vi "S4GUI_003.vi"(7 "Tab ObsEng":enum32{"Obs", "CCD modes", "Guider", "Eng"}(tab)) -> ()   [LabVIEW 2018] (continued)
      n64 = property on="Project ID" class="Str"(error in=w86, "Value"="" ("Observer"), "Text.BGColor"=u32 16448250) -> ()  [unwired: 1 in, 2 out]
      n65 = property on="SendExpose" class="Bool (strict)"(error in=w86, "Value"=TRUE ("ExtSync")) -> ()  [unwired: 1 in, 2 out]
      n66 = property on="suffix alert" class="Str"(error in=w86, "Text.BGColor"=u32 16711680, "Text.TextColor"=u32 16776722) -> ()  [unwired: 1 in, 2 out]
      n67 = property on="Object_dflat" class="Str"(error in=w86, "DisabledEnum"=w95) -> ()  [unwired: 1 in, 2 out]
      n68 = property on="Object_zero" class="Str"(error in=w86, "DisabledEnum"=w95) -> ()  [unwired: 1 in, 2 out]
      n69 = property on="Object_sflat" class="Str"(error in=w86, "DisabledEnum"=w95) -> ()  [unwired: 1 in, 2 out]
      n70 = local write "GUIDER"(FALSE ("GUIDER")) -> ()
      n71 = property on="Exptime ch1" class="DigNum (strict)"("Value"=w72) -> ()  [unwired: 2 in, 2 out]
      n72 = property on="Exptime ch2" class="DigNum (strict)"("Value"=w72) -> ()  [unwired: 2 in, 2 out]
      n73 = property on="Exptime ch3" class="DigNum (strict)"("Value"=w72) -> ()  [unwired: 2 in, 2 out]
      n74 = property on="Exptime ch4" class="DigNum (strict)"("Value"=w72) -> ()  [unwired: 2 in, 2 out]
      n75 = property on="dark suffix" class="Str"(error in=w82, "Text.BGColor"=u32 16448250) -> ()  [unwired: 1 in, 2 out]
      n76 = property on="object suffix" class="Str"(error in=w82, "Text.BGColor"=u32 16448250) -> (error out=w76:errorcluster)  [unwired: 1 in, 1 out]
      n77 = property on="dflat suffix" class="Str"(error in=w82, "Text.BGColor"=u32 16448250) -> ()  [unwired: 1 in, 2 out]
      n78 = property on="SET Temp message" class="Bool (strict)"(error in=w76, "Value"=TRUE ("SET Temp message")) -> (error out=w71:errorcluster)  [unwired: 1 in, 1 out]
      n79 = local write "TEST Comments"("Acquisition for testing purposes" ("TEST Comments")) -> ()
      n80 = local write "test suffix"("test" ("test suffix")) -> ()
      n81 = local write "Object_test"("TEST OBJECT" ("Object_test")) -> ()
      n82 = property on="sflat suffix" class="Str"(error in=w76, "Text.BGColor"=u32 16448250) -> ()  [unwired: 1 in, 2 out]
      n83 = property on="zero suffix" class="Str"(error in=w76, "Text.BGColor"=u32 16448250) -> ()  [unwired: 1 in, 2 out]
      n84 = property on="focus suffix" class="Str"(error in=w76, "Text.BGColor"=u32 16448250) -> ()  [unwired: 1 in, 2 out]
      "suffix alert" <- "Invalid char!" ("suffix alert")
      "FT warning" <- "" ("FT warning")
    }
    frame #4 {
      w97 = u32 1 ("# Cycles")
      n85 = local write "# Cycles"(w97) -> ()
      n86 = local write "#cycles ch1"(w97) -> ()
      n87 = local write "#cycles ch2"(w97) -> ()
      n88 = local write "#cycles ch3"(w97) -> ()
      n89 = local write "#cycles ch4"(w97) -> ()
      n90 = local write "Exp ch1"(w97) -> ()
      n91 = local write "Exp ch2"(w97) -> ()
      n92 = local write "Exp ch3"(w97) -> ()
      n93 = local write "Exp ch4"(w97) -> ()
    }
  }
  n94 = disable-structure shown="Enabled" {
    disable-tunnel: "S4ACS_GUI.lvclass" -> [w106 w108]
    disable-tunnel: w5 -> [w105 w107]
    disable-tunnel: [w100 w108] -> w25
    disable-tunnel: [w99 w107] -> w24
    frame Enabled {
      # "Carrega o ultimo filtro escolhido para os 4 canais."
      n95 = local read "Filter1"() -> (w104:u8)
      n96 = local read "Filter2"() -> (w103:u8)
      n97 = local read "Filter3"() -> (w102:u8)
      n98 = local read "Filter4"() -> (w101:u8)
      n99 = call-dynamic "LoadFilters.vi"("Filter 4"=w101, "Filter 3"=w102, "error in (no error)"=w105, "Filter 2"=w103, "Filter 1"=w104, "S4GUI in"=w106) -> ("error out"=w99:errorcluster, "S4GUI out"=w100:refnum<class "S4GUI.lvclass">)  [unwired: 4 in]
    }
    frame Disabled {
    }
  }
  n100 = flat-sequence "Indicadores dos canais da parte inferior da tela principal" {
    frame #0 {
      w109 = ""
      "B1" <- w109
      "PA1" <- w109
      "RO1" <- w109
      "G1" <- w109
      "SI2" <- w109
      "PA2" <- w109
      "G2" <- w109
      "B2" <- w109
      "RO2" <- w109
      "EA2" <- w109
      "SI3" <- w109
      "EA3" <- w109
      "PA3" <- w109
      "B3" <- w109
      "G3" <- w109
      "RO3" <- w109
      "SI4" <- w109
      "EA4" <- w109
      "PA4" <- w109
      "B4" <- w109
      "G4" <- w109
      "RO4" <- w109
      "SI1" <- w109
      "EA1" <- w109
    }
  }
  n101 = call-dynamic "Write GUI version.vi"("error in (no error)"=w24, "GUI version"=w22, "S4GUI in"=w25) -> ("error out"=w16:errorcluster, "S4GUI out"=w23:refnum<class "S4GUI.lvclass">)  [unwired: 7 in]
  n102 = property on="Tab Acq Type" class="TabCtl (strict)"(error in=w16, "DisabledEnum"=T12."Disabled and Grayed Out" ("Disabled")) -> (error out=w15:errorcluster)  [unwired: 1 in, 1 out]
  n103 = control-ref of="Current Configuration"() -> (w33:refnum<vi>)
  n104 = control-ref of="Parameters"() -> (w30:refnum<vi>)
  n105 = call-dynamic "Initialize.vi"("error in (no error)"=w15, "S4ACS_GUI in"=w23) -> ("error out"=w14:errorcluster, "S4ACS_GUI out"=w18:refnum<class "S4GUI.lvclass">)  [unwired: 8 in]
  n106 = property on="Tab Acq Type" class="TabCtl (strict)"(error in=w14, "DisabledEnum"=T12."Enabled" ("Disabled")) -> (error out=w13:errorcluster)  [unwired: 1 in, 1 out]
  n107 = property on="Property Node" class="Clust (strict)"(reference=w30, "Top"=230 ("Position:Top")) -> (reference out=w34:refnum<vi>)  [unwired: 1 in, 1 out]
  n108 = property on="Property Node" class="Clust (strict)"(reference=w33, "Top"=230 ("Position:Top")) -> (reference out=w32:refnum<vi>)  [unwired: 1 in, 1 out]
  n109 = call-dynamic "Read TabAcqType index.vi"("error in (no error)"=w13, "S4GUI in"=w18) -> ("error out"=w10:errorcluster, "TabAcqType index"=w17:u32, "S4GUI out"=w11:refnum<class "S4GUI.lvclass">)  [unwired: 7 in]
  n110 = case shown="1" w17 {
    tunnel: [T1."OBJECT" ("Tab Acq Type") T1."TEST" ("Tab Acq Type") T1."DFLAT" ("Tab Acq Type") T1."SFLAT" ("Tab Acq Type") T1."DARK" ("Tab Acq Type") T1."ZERO" ("Tab Acq Type") T1."FOCUS" ("Tab Acq Type")] -> w7
    frame 0, Default {
    }
    frame 1 {
    }
    frame 2 {
    }
    frame 3 {
    }
    frame 4 {
    }
    frame 5 {
    }
    frame 6 {
    }
  }
  n111 = local write "Tab Acq Type"(w7) -> ()
  n112 = Bundle("Parameters"=w34, "Current Configuration"=w32) -> (w31:T13)  [unwired: 1 in]
  n113 = call-dynamic "Write ExpMode.vi"("error in (no error)"=w10, "ExpMode"=w7, "S4GUI in"=w11) -> ("error out"=w9:errorcluster, "S4GUI out"=w8:refnum<class "S4GUI.lvclass">)  [unwired: 7 in]
  n114 = while {
    shift-right: [w135] -> w4
    shift-left: w8 -> [w137]
    shift-right: [w122] -> w2
    shift-left: w9 -> [w118]
    tunnel: w31 -> [w142]
    i -> [w128]
    stop <- w119 stop-if-true
    # "Sufixo do arquivo SEMPRE\nem minúsculas."
    n115 = case shown="\"TEST\"" "Tab Acq Type" {
      tunnel: ["object suffix" "test suffix" "dflat suffix" "sflat suffix" "dark suffix" "zero suffix" "focus suffix"] -> w130
      tunnel: ["OBJECT Comments" "TEST Comments" "DFLAT Comments" "SFLAT Comments" "DARK Comments" "ZERO Comments" "FOCUS Comments"] -> w143
      tunnel: ["OBJECT" "TEST" "FLAT" "FLAT" "DARK" "ZERO" "FOCUS"] -> w140
      tunnel: ["Object_obj" "Object_test" "DOMEFLAT" "SKYFLAT" "Object_dark" "ZERO" "Object_focus"] -> w139
      tunnel: [_ _ _ _ _ _ "Start focus"] -> w127
      tunnel: [_ _ _ _ _ _ "Step focus"] -> w125
      tunnel: [_ _ _ _ _ _ "#steps"] -> w126
      frame "OBJECT", Default {
      }
      frame "TEST" {
      }
      frame "DFLAT" {
      }
      frame "SFLAT" {
      }
      frame "DARK" {
      }
      frame "ZERO" {
      }
      frame "FOCUS" {
      }
    }
    n116 = flat-sequence {
      tunnel: w137 -> [w157]
      tunnel: [w157] -> w117
      tunnel: [w156] -> w134
      frame #0 {
        n117 = case shown="False" "reset max" {
          frame False {
          }
          frame True {
            n118 = local write "loop max(ms)"(u32 0 ("loop max(ms)")) -> ()
          }
        }
        n119 = Tick Count (ms)() -> (millisecond timer value=w156:u32)
      }
    }
    n120 = To Lower Case(string=w130) -> (all lower case string=w129:string)
    n121 = event shown="[57] \"#cycles ch4\": Value Change" {
      selector: _ -> [_ _ _ _ _ _ _ _ _ _ _ _ _ _ _ _ _ _ _ _ _ _ _ _ _ _ _ _ _ _ _ _ _ _ _ _ _ _ _ _ _ _ _ _ _ _ _ _ _ _ _ _ _ _ _ _ _ _ _ _ _ _ _ _ _ _ _ _ _ _ _ _ _ _ _ _ _ _ _ _ _ _ _ _ _ _ _ _ _ _ _ _ _ _ _ _ _ _ _ _ _ _ _ _ _ _ _ _ _ _ _ _ _ _ _ _ _ _ _ _ _ _ _ _ _ _ _ _ _ _ _ _ _ _ _ _ _ _ _ _ _ _ _ _ _]
      dyn-events: _ -> [_ _ _ _ _ _ _ _ _ _ _ _ _ _ _ _ _ _ _ _ _ _ _ _ _ _ _ _ _ _ _ _ _ _ _ _ _ _ _ _ _ _ _ _ _ _ _ _ _ _ _ _ _ _ _ _ _ _ _ _ _ _ _ _ _ _ _ _ _ _ _ _ _ _ _ _ _ _ _ _ _ _ _ _ _ _ _ _ _ _ _ _ _ _ _ _ _ _ _ _ _ _ _ _ _ _ _ _ _ _ _ _ _ _ _ _ _ _ _ _ _ _ _ _ _ _ _ _ _ _ _ _ _ _ _ _ _ _ _ _ _ _ _ _ _]
      timeout: 20 -> [_ _ _ _ _ _ _ _ _ _ _ _ _ _ _ _ _ _ _ _ _ _ _ _ _ _ _ _ _ _ _ _ _ _ _ _ _ _ _ _ _ _ _ _ _ _ _ _ _ _ _ _ _ _ _ _ _ _ _ _ _ _ _ _ _ _ _ _ _ _ _ _ _ _ _ _ _ _ _ _ _ _ _ _ _ _ _ _ _ _ _ _ _ _ _ _ _ _ _ _ _ _ _ _ _ _ _ _ _ _ _ _ _ _ _ _ _ _ _ _ _ _ _ _ _ _ _ _ _ _ _ _ _ _ _ _ _ _ _ _ _ _ _ _ _]
      tunnel: w117 -> [w199 w1995 w2006 w2011 w2016 w2021 w2026 w2031 w2301 w2460 w2490 w2496 w2518 w2540 w2739 w2747 w2826 w2847 w2919 w2990 w3091 w3105 w3246 w3485 w3517 w3549 w3581 w3616 w3651 w3686 w3721 w3724 w3819 w4024 w4085 w4612 w4691 w4763 w4834 w4907 w4958 w4999 w5441 w5447 w5567 w6952 w7095 w7300 w7488 w7752 w7971 w7986 w8197 w8407 w8431 w8455 w8479 w8503 w8518 w8660 w8802 w8931 w8951 w8971 w8991 w9012 w9077 w9142 w9207 w9272 w9309 w9337 w9365 w9394 w9467 w9597 w9631 w9690 w9749 w9808 w9867 w9887 w9914 w9930 w9951 w9981 w10011 w10036 w10077 w10118 w10159 w10200 w10241 w10282 w10323 w10366 w10481 w10591 w10701 w10810 w10820 w10840 w10855 w10870 w10885 w10900 w10915 w10930 w10945 w10976 w11005 w11029 w11071 w11105 w11132 w11155 w11183 w11203 w11218 w11238 w11321 w11649 w11675 w11841 w11861 w11876 w11892 w11912 w11932 w11952 w11972 w11987 w12003 w12023 w12043 w12063 w12083 w12098 w12118 w12138 w12158 w12173 w12193 w12213 w12233]
      tunnel: w118 -> [w198 w1994 w2005 w2010 w2015 w2020 w2025 w2030 w2302 w2458 w2489 w2495 w2517 w2539 w2738 w2746 w2825 w2846 w2918 w2991 w3090 w3097 w3242 w3484 w3516 w3548 w3580 w3615 w3650 w3685 w3720 w3732 w3820 w4023 w4084 w4611 w4690 w4762 w4830 w4906 w4956 w4998 w5397 w5446 w5566 w6951 w7094 w7299 w7487 w7745 w7969 w7985 w8195 w8406 w8430 w8454 w8478 w8502 w8517 w8658 w8801 w8932 w8952 w8972 w8992 w9011 w9076 w9141 w9206 w9270 w9307 w9335 w9363 w9393 w9466 w9596 w9630 w9689 w9748 w9807 w9866 w9886 w9913 w9929 w9950 w9980 w10010 w10035 w10076 w10117 w10158 w10199 w10240 w10281 w10322 w10365 w10480 w10590 w10700 w10809 w10819 w10839 w10854 w10869 w10884 w10899 w10914 w10929 w10944 w10975 w11004 w11028 w11070 w11104 w11131 w11154 w11182 w11202 w11217 w11237 w11322 w11648 w11674 w11840 w11860 w11875 w11891 w11911 w11931 w11951 w11971 w11986 w12002 w12022 w12042 w12062 w12082 w12097 w12117 w12137 w12157 w12172 w12192 w12212 w12232]
      tunnel: [w195 w1993 w2003 w2007 w2012 w2017 w2022 w2027 w2264 w2452 w2477 w2497 w2519 w2541 w2726 w2764 w2825 w2864 w2936 w3008 w3077 w3103 w3244 w3395 w3503 w3535 w3567 w3606 w3641 w3676 w3711 w3732 w3740 w3942 w4072 w4531 w4688 w4760 w4825 w4904 w4959 w4993 w5400 w5443 w5534 w7009 w7088 w7293 w7499 w7746 w7970 w7978 w8183 w8329 w8413 w8438 w8462 w8486 w8504 w8647 w8787 w8930 w8950 w8970 w8990 w9010 w9075 w9140 w9205 w9271 w9308 w9336 w9364 w9398 w9471 w9598 w9629 w9688 w9747 w9806 w9865 w9885 w9912 w9928 w9949 w9979 w10009 w10038 w10079 w10120 w10161 w10202 w10243 w10284 w10325 w10364 w10479 w10589 w10699 w10806 w10818 w10838 w10853 w10868 w10883 w10898 w10913 w10928 w10943 w10960 w11002 w11027 w11069 w11103 w11130 w11153 w11165 w11185 w11205 w11221 w11245 w11656 w11679 w11823 w11843 w11863 w11884 w11897 w11917 w11934 w11954 w11974 w11991 w12006 w12026 w12045 w12065 w12085 w12101 w12120 w12140 w12160 w12176 w12195 w12215] -> w122
      tunnel: [w196 _ _ _ _ _ _ _ _ _ _ _ _ _ _ _ _ _ _ _ _ _ _ _ _ _ _ _ _ _ _ _ _ _ _ _ _ _ _ _ _ _ _ _ _ _ _ _ _ _ _ _ _ _ _ _ _ _ _ _ _ _ _ _ _ _ _ _ _ _ _ _ _ _ _ _ _ _ _ _ _ _ _ _ _ _ _ _ _ _ _ _ _ _ _ _ _ _ _ _ _ _ _ _ _ _ _ _ _ _ _ _ _ _ _ _ _ _ _ _ _ _ _ _ _ _ _ _ _ _ _ _ _ _ _ _ _ _ _ _ _ _ _ _ _] -> w120
      tunnel: w129 -> [_ _ _ _ _ _ _ _ _ _ _ _ _ _ _ _ _ _ _ _ _ _ _ _ _ _ _ _ _ _ _ _ _ _ _ _ _ _ _ _ _ w4992 _ _ _ _ w7093 w7297 _ w7750 _ w7983 w8204 _ _ _ _ _ w8525 w8667 w8809 _ _ _ _ _ _ _ _ _ _ _ _ _ _ _ _ _ _ _ _ _ _ _ _ _ _ _ _ _ _ _ _ _ _ _ _ _ _ _ _ _ _ _ _ _ _ _ _ _ _ _ _ _ _ _ _ _ _ _ _ _ _ _ _ _ _ _ _ _ _ _ _ _ _ _ _ _ _ _ _ _ _ _ _]
      tunnel: w143 -> [_ _ _ _ _ _ _ _ _ _ _ _ _ _ _ _ _ _ _ _ _ _ _ _ _ _ _ _ _ _ _ _ _ _ _ _ _ _ _ _ _ w4991 _ _ _ _ w7092 _ w7503 w7749 _ w7982 w8203 _ _ _ _ _ w8524 w8666 w8808 _ _ _ _ _ _ _ _ _ _ _ _ _ _ _ _ _ _ _ _ _ _ _ _ _ _ _ _ _ _ _ _ _ _ _ _ _ _ _ _ _ _ _ _ _ _ _ _ _ _ _ _ _ _ _ _ _ _ _ _ _ _ _ _ _ _ _ _ _ _ _ _ _ _ _ _ _ _ _ _ _ _ _ _]
      tunnel: w142 -> [_ _ _ _ _ _ _ _ _ _ _ _ _ _ _ _ _ _ _ _ _ _ _ _ _ _ _ _ _ _ _ w3725 _ _ _ _ _ _ _ _ _ _ _ _ _ _ _ _ _ _ _ _ _ _ _ _ _ _ _ _ _ _ _ _ _ _ _ _ _ _ _ _ _ _ _ _ _ _ _ _ _ _ _ _ _ _ _ _ _ _ _ _ _ _ _ _ _ _ _ _ _ _ _ _ _ _ _ _ _ _ _ _ _ _ _ _ _ _ _ _ _ _ _ _ _ _ _ _ _ _ _ _ _ _ _ _ _ _ _ _ _ _ _ _ _]
      tunnel: [w194 w1995 w2004 w2008 w2013 w2018 w2023 w2028 w2266 w2451 w2478 w2498 w2520 w2542 w2727 w2765 w2826 w2865 w2937 w3009 w3068 w3104 w3245 w3397 w3494 w3526 w3558 w3583 w3618 w3653 w3688 w3724 w3741 w3939 w4073 w4532 w4689 w4761 w4826 w4905 w4960 w4973 w5401 w5442 w5535 w7008 w7089 w7294 w7500 w7747 w7971 w7979 w8184 w8330 w8414 w8439 w8463 w8487 w8505 w8646 w8789 w8929 w8949 w8969 w8989 w9009 w9074 w9139 w9204 w9269 w9306 w9334 w9362 w9396 w9469 w9599 w9628 w9687 w9746 w9805 w9864 w9884 w9904 w9927 w9948 w9978 w10008 w10037 w10078 w10119 w10160 w10201 w10242 w10283 w10324 w10363 w10478 w10588 w10698 w10807 w10811 w10834 w10849 w10864 w10879 w10894 w10909 w10924 w10939 w10959 w10977 w11014 w11038 w11086 w11116 w11141 w11164 w11184 w11204 w11219 w11246 w11657 w11680 w11822 w11842 w11862 w11883 w11895 w11915 w11933 w11953 w11973 w11990 w12004 w12024 w12044 w12064 w12084 w12099 w12119 w12139 w12159 w12174 w12194 w12214] -> w136
      tunnel: "Input Cluster" -> [_ _ _ _ _ _ _ _ _ _ _ _ _ _ _ _ _ _ _ _ _ _ _ _ _ _ _ _ _ _ _ w3723 _ _ _ _ _ _ _ _ _ _ _ _ _ _ _ _ _ _ _ _ _ _ _ _ _ _ _ _ _ _ _ _ _ _ _ _ _ _ _ _ _ _ _ _ _ _ _ _ _ _ _ _ _ _ _ _ _ _ _ _ _ _ _ _ _ _ _ _ _ _ _ _ _ _ _ _ _ _ _ _ _ _ _ _ _ _ _ _ _ _ _ _ _ _ _ _ _ _ _ _ _ _ _ _ _ _ _ _ _ _ _ _ _]
      tunnel: w140 -> [_ _ _ _ _ _ _ _ _ _ _ _ _ _ _ _ _ _ _ _ _ _ _ _ _ _ _ _ _ _ _ _ _ _ _ _ _ _ _ _ _ w4990 _ _ _ _ w7090 w7295 w7501 w7748 _ w7980 w8202 _ _ _ _ _ w8523 w8664 w8807 _ _ _ _ _ _ _ _ _ _ _ _ _ _ _ _ _ _ _ _ _ _ _ _ _ _ _ _ _ _ _ _ _ _ _ _ _ _ _ _ _ _ _ _ _ _ _ _ _ _ _ _ _ _ _ _ _ _ _ _ _ _ _ _ _ _ _ _ _ _ _ _ _ _ _ _ _ _ _ _ _ _ _ _]
      tunnel: w139 -> [_ _ _ _ _ _ _ _ _ _ _ _ _ _ _ _ _ _ _ _ _ _ _ _ _ _ _ _ _ _ _ _ _ _ _ _ _ _ _ _ _ w4989 _ _ _ _ _ w7298 w7504 w7751 _ w7984 w8201 _ _ _ _ _ w8522 w8665 w8806 _ _ _ _ _ _ _ _ _ _ _ _ _ _ _ _ _ _ _ _ _ _ _ _ _ _ _ _ _ _ _ _ _ _ _ _ _ _ _ _ _ _ _ _ _ _ _ _ _ _ _ _ _ _ _ _ _ _ _ _ _ _ _ _ _ _ _ _ _ _ _ _ _ _ _ _ _ _ _ _ _ _ _ _]
      tunnel: "Observer" -> [_ _ _ _ _ _ _ _ _ _ _ _ _ _ _ _ _ _ _ _ _ _ _ _ _ _ _ _ _ _ _ _ _ _ _ _ _ _ _ _ _ w4988 _ _ w5540 w6961 w7091 w7296 w7502 _ _ w7981 w8200 _ _ _ _ _ w8521 w8663 w8805 _ _ _ _ _ _ _ _ _ _ _ _ _ _ _ _ _ _ _ _ _ _ _ _ _ _ _ _ _ _ _ _ _ _ _ _ _ _ _ _ _ _ _ _ _ _ _ _ _ _ _ _ _ _ _ _ _ _ _ _ _ _ _ _ _ _ _ _ _ _ _ _ _ _ _ _ _ _ _ _ _ _ _ _]
      tunnel: w128 -> [w197 _ _ _ _ _ _ _ _ _ _ _ _ _ _ _ _ _ _ _ _ _ _ _ _ _ _ _ _ _ _ _ _ _ _ _ _ _ _ _ _ _ _ _ _ _ _ _ _ _ _ _ _ _ _ _ _ _ _ _ _ _ _ _ _ _ _ _ _ _ _ _ _ _ _ _ _ _ _ _ _ _ _ _ _ _ _ _ _ _ _ _ _ _ _ _ _ _ _ _ _ _ _ _ _ _ _ _ _ _ _ _ _ _ _ _ _ _ _ _ _ _ _ _ _ _ _ _ _ _ _ _ _ _ _ _ _ _ _ _ _ _ _ _ _]
      tunnel: "Tab Acq Type" -> [_ _ _ _ _ _ _ _ _ _ _ _ _ _ _ _ _ _ _ _ _ _ _ _ _ _ _ _ _ _ _ _ _ _ _ _ _ _ _ _ _ w4980 _ _ _ _ _ _ w7490 _ _ _ w8191 _ _ _ _ _ w8512 w8654 w8795 _ _ _ _ _ _ _ _ _ _ _ _ _ _ _ _ _ _ _ _ _ _ _ _ _ _ _ _ _ _ _ _ _ _ _ _ _ _ _ _ _ _ _ _ _ _ _ _ _ _ _ _ _ _ _ _ _ _ _ _ _ _ _ _ _ _ _ _ _ _ _ _ _ _ _ _ _ _ _ _ _ _ _ _]
      tunnel: w127 -> [_ _ _ _ _ _ _ _ _ _ _ _ _ _ _ _ _ _ _ _ _ _ _ _ _ _ _ _ _ _ _ _ _ _ _ _ _ _ _ _ _ w4979 _ _ _ _ _ _ _ _ _ _ w8190 _ _ _ _ _ w8511 w8653 w8794 _ _ _ _ _ _ _ _ _ _ _ _ _ _ _ _ _ _ _ _ _ _ _ _ _ _ _ _ _ _ _ _ _ _ _ _ _ _ _ _ _ _ _ _ _ _ _ _ _ _ _ _ _ _ _ _ _ _ _ _ _ _ _ _ _ _ _ _ _ _ _ _ _ _ _ _ _ _ _ _ _ _ _ _]
      tunnel: w126 -> [_ _ _ _ _ _ _ _ _ _ _ _ _ _ _ _ _ _ _ _ _ _ _ _ _ _ _ _ _ _ _ _ _ _ _ _ _ _ _ _ _ w4977 _ _ _ _ _ _ _ _ _ _ w8188 _ _ _ _ _ w8509 w8651 w8792 _ _ _ _ _ _ _ _ _ _ _ _ _ _ _ _ _ _ _ _ _ _ _ _ _ _ _ _ _ _ _ _ _ _ _ _ _ _ _ _ _ _ _ _ _ _ _ _ _ _ _ _ _ _ _ _ _ _ _ _ _ _ _ _ _ _ _ _ _ _ _ _ _ _ _ _ _ _ _ _ _ _ _ _]
      tunnel: w125 -> [_ _ _ _ _ _ _ _ _ _ _ _ _ _ _ _ _ _ _ _ _ _ _ _ _ _ _ _ _ _ _ _ _ _ _ _ _ _ _ _ _ w4978 _ _ _ _ _ _ _ _ _ _ w8189 _ _ _ _ _ w8510 w8652 w8793 _ _ _ _ _ _ _ _ _ _ _ _ _ _ _ _ _ _ _ _ _ _ _ _ _ _ _ _ _ _ _ _ _ _ _ _ _ _ _ _ _ _ _ _ _ _ _ _ _ _ _ _ _ _ _ _ _ _ _ _ _ _ _ _ _ _ _ _ _ _ _ _ _ _ _ _ _ _ _ _ _ _ _ _]
      tunnel: "Project ID" -> [_ _ _ _ _ _ _ _ _ _ _ _ _ _ _ _ _ _ _ _ _ _ _ _ _ _ _ _ _ _ _ _ _ _ _ _ _ _ _ _ _ _ _ _ w5539 w6960 _ _ _ _ _ _ _ _ _ _ _ _ _ _ _ _ _ _ _ _ _ _ _ _ _ _ _ _ _ _ _ _ _ _ _ _ _ _ _ _ _ _ _ _ _ _ _ _ _ _ _ _ _ _ _ _ _ _ _ _ _ _ _ _ _ _ _ _ _ _ _ _ _ _ _ _ _ _ _ _ _ _ _ _ _ _ _ _ _ _ _ _ _ _ _ _ _ _ _]
      event Timeout {
        # "execução do botão\nOK do SET TEMP de\ntodos os canais."
        # "2024.07.02: Mostra as publicações das aplicações."
        # "Trata as tarefas para atender \naos clientes: Publisher"
        # "Conteudo dos indicadores"
        # "Status dos indicadores: Habilitado ou Desab."
        # "Obtém os valores de status dos\ndispositivos de cada servidor para\napresentar nos indicadores da GUI."
        # "Trata as tarefas individuais de \ncada servidor (ACS1,...,ACS4, \nICS, TCS, Focus,Weather)"
        # "Determina a sequência de\ntarefas dos servidores\npara uma observação, de \nacordo com o modo de \noperação (disparado com \nos botões START)"
        # "execução dos botões\n no modo sincrono."
        # "execução dos botões\n no modo assincrono."
        n122 = event-data() -> ()  [unwired: 1 in, 2 out]
        n123 = disable-structure shown="Enabled" {
          disable-tunnel: w199 -> [w236 _]
          disable-tunnel: w198 -> [w234 _]
          frame Disabled {
            n124 = flat-sequence {
              tunnel: [w245] -> w235
              tunnel: w236 -> [w245]
              tunnel: w234 -> [w244]
              tunnel: [w244] -> w233
              frame #0 {
                n125 = local read "time alert"() -> (w242:u32)
                n126 = Tick Count (ms)() -> (millisecond timer value=w243:u32)
                n127 = Subtract(x=w243, y=w242) -> (x-y=w241:u32)
                n128 = Greater?(x=w241, y=u32 750) -> (0:w239:bool)
                n129 = case shown="True" w239 {
                  frame False {
                  }
                  frame True {
                    n130 = property on="suffix alert" class="Str"("Visible"=FALSE) -> ()  [unwired: 2 in, 2 out]
                  }
                }
              }
            }
            n131 = local read "charKeyboardInteger"() -> (w237:i16)
            n132 = call-dynamic "Read ExpMode.vi"("error in (no error)"=w233, "S4GUI in"=w235) -> ("ExpMode"=w238:T1)  [unwired: 7 in, 2 out]
            n133 = case shown="Default" w237 {
              tunnel: w238 -> [_ w247 w269]
              frame 32767 {
              }
              frame 0, 8, 32, 48..57, 65..90, 97..122 {
                n134 = case shown="\"OBJECT\", Default" w247 {
                  tunnel: [w252 w253 w254 w255 w256 w257] -> w248
                  frame "OBJECT", Default {
                    n135 = local read "object suffix"() -> (w252:string)
                  }
                  frame "DFLAT" {
                    n136 = local read "dflat suffix"() -> (w253:string)
                  }
                  frame "SFLAT" {
                    n137 = local read "sflat suffix"() -> (w254:string)
                  }
                  frame "DARK" {
                    n138 = local read "dark suffix"() -> (w255:string)
                  }
                  frame "ZERO" {
                    n139 = local read "zero suffix"() -> (w256:string)
                  }
                  frame "FOCUS" {
                    n140 = local read "focus suffix"() -> (w257:string)
                  }
                }
                n141 = String Length(string=w248) -> (length=w251:i32)
                n142 = Greater?(x=w251, y=10) -> (0:w249:bool)
                n143 = case shown="True" w249 {
                  tunnel: w248 -> [w258 _]
                  tunnel: w247 -> [_ w260]
                  frame False {
                    n144 = local write "suffix temp"(w258) -> ()
                  }
                  frame True {
                    n145 = local read "suffix temp"() -> (w259:string)
                    n146 = case shown="\"OBJECT\", Default" w260 {
                      tunnel: w259 -> [w261 w262 w263 w264 w265 w266]
                      frame "OBJECT", Default {
                        n147 = local write "object suffix"(w261) -> ()
                      }
                      frame "DFLAT" {
                        n148 = local write "dflat suffix"(w262) -> ()
                      }
                      frame "SFLAT" {
                        n149 = local write "sflat suffix"(w263) -> ()
                      }
                      frame "DARK" {
                        n150 = local write "dark suffix"(w264) -> ()
                      }
                      frame "ZERO" {
                        n151 = local write "zero suffix"(w265) -> ()
                      }
                      frame "FOCUS" {
                        n152 = local write "focus suffix"(w266) -> ()
                      }
                    }
                  }
                }
              }
              frame Default {
                n153 = local write "charKeyboardInteger"(i16 32767 ("lastChar")) -> ()
                n154 = Tick Count (ms)() -> (millisecond timer value=→"time alert":u32)
                n155 = property on="suffix alert" class="Str"("Visible"=TRUE) -> ()  [unwired: 2 in, 2 out]
                n156 = case shown="\"OBJECT\", Default" w269 {
                  tunnel: "suffix temp" -> [w272 w273 w274 w275 w276 w277]
                  frame "OBJECT", Default {
                    n157 = local write "object suffix"(w272) -> ()
                  }
                  frame "DFLAT" {
                    n158 = local write "dflat suffix"(w273) -> ()
                  }
                  frame "SFLAT" {
                    n159 = local write "sflat suffix"(w274) -> ()
                  }
                  frame "DARK" {
                    n160 = local write "dark suffix"(w275) -> ()
                  }
                  frame "ZERO" {
                    n161 = local write "zero suffix"(w276) -> ()
                  }
                  frame "FOCUS" {
                    n162 = local write "focus suffix"(w277) -> ()
                  }
                }
              }
            }
          }
          frame Enabled {
          }
        }
        n163 = disable-structure shown="Enabled" {
          disable-tunnel: w199 -> [w283 w288]
          disable-tunnel: w198 -> [w282 w286]
          disable-tunnel: [w280 w285] -> w191
          disable-tunnel: [w279 w284] -> w193
          disable-tunnel: w197 -> [_ w287]
          frame Disabled {
            n164 = call "Elapsed Time"() -> ("Time has Elapsed"=w278:bool)  [unwired: 12 in, 7 out]
            n165 = call "Elapsed Time3"() -> ("Time has Elapsed"=w281:bool)  [unwired: 12 in, 7 out]
            n166 = call "Write Status_timeout.vi"("error in (no error)"=w282, "TCS_timeout"=w281, "Status_timeout"=w278, "S4ACS_GUI in"=w283) -> ("error out"=w280:errorcluster, "S4ACS_GUI out"=w279:refnum<class "S4GUI.lvclass">)  [unwired: 6 in]
          }
          frame Enabled {
            n167 = call-dynamic "Write loop counter.vi"("error in (no error)"=w286, "loop counter"=w287, "S4GUI in"=w288) -> ("error out"=w285:errorcluster, "S4GUI out"=w284:refnum<class "S4GUI.lvclass">)  [unwired: 7 in]
          }
        }
        n168 = call-dynamic "HandleSetTemp.vi"("error in (no error)"=w191, "S4GUI in"=w193) -> ("error out"=w190:errorcluster, "S4GUI out"=w192:refnum<class "S4GUI.lvclass">)  [unwired: 8 in]
        n169 = call-dynamic "GetPubs.vi"("error in (no error)"=w190, "S4GUI in"=w192) -> ("error out"=w210:errorcluster, "Pubs out"=→"All Pubs":T11, "S4GUI out"=w209:refnum<class "S4GUI.lvclass">)  [unwired: 7 in]
        n170 = call-dynamic "HandlePauseAsync.vi"("error in (no error)"=w210, "S4GUI in"=w209) -> ("error out"=w227:errorcluster, "S4GUI out"=w229:refnum<class "S4GUI.lvclass">)  [unwired: 8 in]
        n171 = call-dynamic "HandleStopAsync.vi"("error in (no error)"=w227, "S4GUI in"=w229) -> ("error out"=w226:errorcluster, "S4GUI out"=w228:refnum<class "S4GUI.lvclass">)  [unwired: 8 in]
        n172 = call-dynamic "HandleAbortAsync.vi"("error in (no error)"=w226, "S4GUI in"=w228) -> ("error out"=w220:errorcluster, "S4GUI out"=w221:refnum<class "S4GUI.lvclass">)  [unwired: 8 in]
        n173 = call-dynamic "HandlePauseSync.vi"("error in (no error)"=w220, "S4GUI in"=w221) -> ("error out"=w219:errorcluster, "S4GUI out"=w218:refnum<class "S4GUI.lvclass">)  [unwired: 8 in]
        n174 = call-dynamic "HandleStopSync.vi"("error in (no error)"=w219, "S4GUI in"=w218) -> ("error out"=w223:errorcluster, "S4GUI out"=w225:refnum<class "S4GUI.lvclass">)  [unwired: 8 in]
        n175 = call-dynamic "HandleAbortSync.vi"("error in (no error)"=w223, "S4GUI in"=w225) -> ("error out"=w222:errorcluster, "S4GUI out"=w224:refnum<class "S4GUI.lvclass">)  [unwired: 8 in]
        n176 = call-dynamic "HandleObservation.vi"("error in (no error)"=w222, "S4ACS_GUI in"=w224) -> ("error out"=w231:errorcluster, "S4ACS_GUI out"=w232:refnum<class "S4GUI.lvclass">)  [unwired: 8 in]
        n177 = call-dynamic "HandleServers.vi"("error in (no error)"=w231, "S4GUI in"=w232) -> ("error out"=w213:errorcluster, "S4GUI out"=w214:refnum<class "S4GUI.lvclass">)  [unwired: 8 in]
        n178 = call-dynamic "HandleClients.vi"("error in (no error)"=w213, "S4GUI in"=w214) -> ("error out"=w212:errorcluster, "S4GUI out"=w204:refnum<class "S4GUI.lvclass">)  [unwired: 8 in]
        n179 = call-dynamic "GetStatus.vi"("error in (no error)"=w212, "S4GUI in"=w204) -> ("error out"=w206:errorcluster, "S4GUI out"=w203:refnum<class "S4GUI.lvclass">)  [unwired: 8 in]
        n180 = call-dynamic "Read output cluster.vi"("error in (no error)"=w206, "S4GUI in"=w203) -> ("error out"=w205:errorcluster, "output cluster"=w200:T15, "S4GUI out"=w202:refnum<class "S4GUI.lvclass">)  [unwired: 7 in]
        n181 = call "Elapsed Time2"() -> ("Time has Elapsed"=w217:bool)  [unwired: 12 in, 7 out]
        n182 = call-dynamic "Read Cluster Disable.vi"("error in (no error)"=w205, "S4GUI in"=w202) -> ("error out"=w207:errorcluster, "Cluster Disable"=w208:T16, "S4GUI out"=w201:refnum<class "S4GUI.lvclass">)  [unwired: 7 in]
        n183 = call "Read cfg file.vi"("error in (no error)"=w207, "S4ACS_GUI in"=w201) -> ("error out"=w215:errorcluster, "cfg file"=w230:string, "S4ACS_GUI out"=w216:refnum<class "S4GUI.lvclass">)  [unwired: 7 in]
        n184 = case shown="True" w217 {
          tunnel: w200 -> [_ w346]
          tunnel: w208 -> [_ w345]
          tunnel: w230 -> [_ w344]
          tunnel: w216 -> [w291 w343]
          tunnel: w215 -> [w290 w342]
          tunnel: [w290 w294] -> w195
          tunnel: [FALSE ("exit") w293] -> w196
          tunnel: [w291 w292] -> w194
          frame False {
          }
          frame True {
            w301 = "arking" ("regular expression")
            w319 = "ERRO" ("regular expression")
            # "Verifica mudança de modo e se deve carregar valores default \npara procedimento de ajuste de foco do telescópio."
            # "1a vez FOTOM (F)"
            # "1a vez POLAR (F)"
            # "MODE:\nF -> photometric\nT -> polarimetric"
            n185 = stacked-sequence {
              tunnel: w343 -> [w395 w402 w413 w423 w432]
              tunnel: w342 -> [w394 w401 w412 w422 w431]
              tunnel: [_ _ _ _ w430] -> w336
              tunnel: [_ _ _ _ w429] -> w335
              tunnel: [_ _ _ _ w428] -> w304
              frame #0 {
                n186 = call-dynamic "Read AcquisitionA.vi"("error in (no error)"=w394, "S4ACS_GUI in"=w395) -> ("error out"=w391:errorcluster, "Acquisition.lvclass"=w393:refnum<class "Acquisition.lvclass">)  [unwired: 7 in, 1 out]
                n187 = call-dynamic "Read Channel.vi"("error in (no error)"=w391, "Acquisition in"=w393) -> ("error out"=w390:errorcluster, "Channel.lvclass"=w392:refnum<class "Channel.lvclass">)  [unwired: 7 in, 1 out]
                n188 = call-dynamic "Read CyclesDone.vi"("error in (no error)"=w390, "Channel in"=w392) -> ("error out"=→"error out 6":errorcluster, "CyclesDone"=w387:u32)  [unwired: 7 in, 1 out]
                "Cycles Done ch1" <- w387
                n189 = Number To Decimal String(number=w387) -> (decimal integer string=w386:string)  [unwired: 1 in]
                n190 = Concatenate Strings("#Cycles Done ", w386) -> (w385:string)
                n191 = property on="Cycles Done ch1" class="Slide (strict)"("Caption.Text"=w385) -> ()  [unwired: 2 in, 2 out]
              }
              frame #1 {
                n192 = call "Read AcquisitionB.vi"("error in (no error)"=w401, "S4ACS_GUI in"=w402) -> ("error out"=w404:errorcluster, "Acquisition.lvclass"=w405:refnum<class "Acquisition.lvclass">)  [unwired: 7 in, 1 out]
                n193 = call-dynamic "Read Channel.vi"("error in (no error)"=w404, "Acquisition in"=w405) -> ("error out"=w403:errorcluster, "Channel.lvclass"=w406:refnum<class "Channel.lvclass">)  [unwired: 7 in, 1 out]
                n194 = call-dynamic "Read CyclesDone.vi"("error in (no error)"=w403, "Channel in"=w406) -> ("error out"=→"error out 4":errorcluster, "CyclesDone"=w397:u32)  [unwired: 7 in, 1 out]
                "Cycles Done ch2" <- w397
                n195 = Number To Decimal String(number=w397) -> (decimal integer string=w398:string)  [unwired: 1 in]
                n196 = Concatenate Strings("#Cycles Done ", w398) -> (w396:string)
                n197 = property on="Cycles Done ch2" class="Slide (strict)"("Caption.Text"=w396) -> ()  [unwired: 2 in, 2 out]
              }
              frame #2 {
                n198 = call-dynamic "Read AcquisitionC.vi"("error in (no error)"=w412, "S4ACS_GUI in"=w413) -> ("error out"=w415:errorcluster, "Acquisition.lvclass"=w416:refnum<class "Acquisition.lvclass">)  [unwired: 7 in, 1 out]
                n199 = call-dynamic "Read Channel.vi"("error in (no error)"=w415, "Acquisition in"=w416) -> ("error out"=w414:errorcluster, "Channel.lvclass"=w417:refnum<class "Channel.lvclass">)  [unwired: 7 in, 1 out]
                n200 = call-dynamic "Read CyclesDone.vi"("error in (no error)"=w414, "Channel in"=w417) -> ("error out"=→"error out 5":errorcluster, "CyclesDone"=w408:u32)  [unwired: 7 in, 1 out]
                "Cycles Done ch3" <- w408
                n201 = Number To Decimal String(number=w408) -> (decimal integer string=w409:string)  [unwired: 1 in]
                n202 = Concatenate Strings("#Cycles Done ", w409) -> (w407:string)
                n203 = property on="Cycles Done ch3" class="Slide (strict)"("Caption.Text"=w407) -> ()  [unwired: 2 in, 2 out]
              }
              frame #3 {
                n204 = call-dynamic "Read AcquisitionD.vi"("error in (no error)"=w422, "S4ACS_GUI in"=w423) -> ("error out"=w425:errorcluster, "Acquisition.lvclass"=w426:refnum<class "Acquisition.lvclass">)  [unwired: 7 in, 1 out]
                n205 = call-dynamic "Read Channel.vi"("error in (no error)"=w425, "Acquisition in"=w426) -> ("error out"=w424:errorcluster, "Channel.lvclass"=w427:refnum<class "Channel.lvclass">)  [unwired: 7 in, 1 out]
                n206 = call-dynamic "Read CyclesDone.vi"("error in (no error)"=w424, "Channel in"=w427) -> ("CyclesDone"=w419:u32)  [unwired: 7 in, 2 out]
                "Cycles Done ch4" <- w419
                n207 = Number To Decimal String(number=w419) -> (decimal integer string=w420:string)  [unwired: 1 in]
                n208 = Concatenate Strings("#Cycles Done ", w420) -> (w418:string)
                n209 = property on="Cycles Done ch4" class="Slide (strict)"("Caption.Text"=w418) -> ()  [unwired: 2 in, 2 out]
              }
              frame #4 {
                n210 = call-dynamic "Read SET request.vi"("error in (no error)"=w431, "S4GUI in"=w432) -> ("error out"=w429:errorcluster, "SET request"=w428:bool, "S4GUI out"=w430:refnum<class "S4GUI.lvclass">)  [unwired: 7 in]
              }
            }
            n211 = stacked-sequence {
              tunnel: w346 -> [w478 w488 w500 w502 w510 w556 w559 w693 w796 w1138 _ _ _ _ _ w1330 w1516 w1679 w1838 w1948]
              tunnel: [_ _ _ _ _ _ _ w691 _ _ _ _ _ _ _ _ _ _ _ _] -> w326
              tunnel: w345 -> [_ w484 _ _ _ _ _ _ _ _ w1165 w1212 w1229 w1246 w1263 _ _ _ _ _]
              tunnel: w344 -> [_ _ _ _ _ _ _ _ _ _ _ _ _ _ _ w1325 _ _ _ _]
              tunnel: w304 -> [_ _ _ _ _ _ _ _ _ _ _ _ _ _ _ _ _ _ _ w1951]
              frame #0 {
                (unwired) u32 240 ("Tab Control Pane Dimension:Width")
                (unwired) u32 300 ("Tab Control Pane Dimension:Height")
                n212 = Unbundle By Name(w478) -> ("GS STATUS cluster.AG"=→"GUIDER":bool, "TCS id"=w444:u32, "TCSPD_connection"=→"TCSPD":bool, "TCS extended"=w475:string, "focus pos"=w440:i32, "weather status"=w438:T17)
                n213 = Unbundle By Name(w438) -> ("outTemp"=→"Outside Temp":string, "pressure"=→"Pressure":string, "outHumidity"=→"Humidity":string, "windSpeed"=→"Wind Speed[Km/h]":string)
                n214 = Number To Decimal String(number=w440) -> (decimal integer string=→"Telescope Focus":string)  [unwired: 1 in]
                n215 = Equal?(x=u32 6 ("Tab Control Pane Dimension:Width"), y=w444) -> (x = y?=w443:bool)
                n216 = Match Pattern(string=w475, regular expression="RA=") -> (after substring=w471:string)  [unwired: 1 in, 3 out]
                n217 = local write "TCS mode"(w443) -> ()
                n218 = Match Pattern(string=w471, regular expression="DEC=") -> (before substring=→"RA":string, after substring=w470:string)  [unwired: 1 in, 2 out]
                n219 = Match Pattern(string=w470, regular expression="EQUINOX=") -> (before substring=→"DEC":string, after substring=w469:string)  [unwired: 1 in, 2 out]
                n220 = Match Pattern(string=w469, regular expression="AIRMASS=") -> (after substring=w465:string)  [unwired: 1 in, 3 out]
                n221 = Match Pattern(string=w465, regular expression="TCSHA=") -> (before substring=→"Air Mass":string, after substring=w464:string)  [unwired: 1 in, 2 out]
                n222 = Match Pattern(string=w464, regular expression="TCSDATE=") -> (before substring=→"Hour Angle":string, after substring=w462:string)  [unwired: 1 in, 2 out]
                n223 = Match Pattern(string=w462, regular expression="TELFOCUS=") -> (before substring=→"Date":string, after substring=w458:string)  [unwired: 1 in, 2 out]
                n224 = Match Pattern(string=w458, regular expression="EXTTEMP=") -> (after substring=w457:string)  [unwired: 1 in, 3 out]
                n225 = Match Pattern(string=w457, regular expression="PRESSURE=") -> (after substring=w456:string)  [unwired: 1 in, 3 out]
                n226 = Match Pattern(string=w456, regular expression="HUMIDITY=") -> (after substring=w448:string)  [unwired: 1 in, 3 out]
                n227 = Match Pattern(string=w448, regular expression="JD=") -> (after substring=w449:string)  [unwired: 1 in, 3 out]
                n228 = disable-structure shown="Enabled" {
                  disable-tunnel: u32 211 ("Tab Control Pane Dimension:Height") -> [w480 _]
                  disable-tunnel: u32 225 ("Tab Control Pane Dimension:Width") -> [w479 _]
                  frame Disabled {
                    n229 = property on="Tab CH1" class="TabCtl (strict)"("PaneHeight"=w480, "PaneWidth"=w479) -> ()  [unwired: 2 in, 2 out]
                    n230 = property on="Tab CH2" class="TabCtl (strict)"("PaneHeight"=w480, "PaneWidth"=w479) -> ()  [unwired: 2 in, 2 out]
                    n231 = property on="Tab CH3" class="TabCtl (strict)"("PaneHeight"=w480, "PaneWidth"=w479) -> ()  [unwired: 2 in, 2 out]
                    n232 = property on="Tab CH4" class="TabCtl (strict)"("PaneHeight"=w480, "PaneWidth"=w479) -> ()  [unwired: 2 in, 2 out]
                  }
                  frame Enabled {
                  }
                }
                n233 = Match Pattern(string=w449, regular expression="SD=") -> (before substring=→"Julian Date":string, after substring=→"Sideral Time":string)  [unwired: 1 in, 2 out]
              }
              frame #1 {
                # "OV 2024 09 04: Depois da criação da aba CCD modes, TODOS os parametros da aba Camera são protegidos por senha, \ninclusive as chaves de habilitação dos canais."
                n234 = Unbundle By Name(w488) -> ("S4ICS id"=w486:u32)
                n235 = Unbundle By Name(w484) -> ("Cluster AdmCCDsetup.param"=w481:T12)
                n236 = Equal?(x=u32 11, y=w486) -> (x = y?=w485:bool)
                n237 = local write "S4ICS protocol"(w485) -> ()
                n238 = case shown="\"Disabled and Grayed Out\"" w481 {
                  tunnel: [_ w490 w494] -> w483
                  frame Default {
                  }
                  frame "Disabled" {
                    n239 = Build Array(u32 4 ("element"), u32 5 ("element"), u32 6 ("element")) -> (w490:u32[])
                  }
                  frame "Disabled and Grayed Out" {
                    n240 = Build Array(u32 4 ("element"), u32 5 ("element"), u32 6 ("element")) -> (w494:u32[])
                  }
                }
                n241 = property on="Trigger\nMode" class="Ring (strict)"("DisabledEnum"=w481) -> ()  [unwired: 2 in, 2 out]
                n242 = property on="Vertical\nShift Speed" class="Ring (strict)"("DisabledEnum"=w481) -> ()  [unwired: 2 in, 2 out]
                n243 = property on="Vertical\nClock Voltage" class="Ring (strict)"("DisabledEnum"=w481) -> ()  [unwired: 2 in, 2 out]
                n244 = To Long Integer(number=w483) -> (32bit integer=w482:i32[])
                n245 = property on="EM Gain" class="DigNum (strict)"("DisabledEnum"=w481) -> ()  [unwired: 2 in, 2 out]
                n246 = property on="Read\nMode" class="Ring (strict)"("DisabledEnum"=w481) -> ()  [unwired: 2 in, 2 out]
                n247 = property on="AQM" class="Enum (strict)"("Disabled Items []"=w482) -> ()  [unwired: 2 in, 2 out]
                n248 = property on="Acquisition\nMode" class="Ring (strict)"("DisabledEnum"=w481) -> ()  [unwired: 2 in, 2 out]
                n249 = property on="A/D \nChannel" class="DigNum (strict)"("DisabledEnum"=w481) -> ()  [unwired: 2 in, 2 out]
                n250 = property on="Readout\nRate" class="Ring (strict)"("DisabledEnum"=w481) -> ()  [unwired: 2 in, 2 out]
                n251 = property on="CCD \nEM Mode" class="Ring (strict)"("DisabledEnum"=w481) -> ()  [unwired: 2 in, 2 out]
                n252 = property on="CCD\nEM Gain" class="DigNum (strict)"("DisabledEnum"=w481) -> ()  [unwired: 2 in, 2 out]
                n253 = property on="Shutter\nTTL" class="Ring (strict)"("DisabledEnum"=w481) -> ()  [unwired: 2 in, 2 out]
                n254 = property on="Shutter\nOpenning Time" class="DigNum (strict)"("DisabledEnum"=w481) -> ()  [unwired: 2 in, 2 out]
                n255 = property on="Frame\nTransfer" class="Bool (strict)"("DisabledEnum"=w481) -> ()  [unwired: 2 in, 2 out]
                n256 = property on="Shutter\nMode" class="Ring (strict)"("DisabledEnum"=w481) -> ()  [unwired: 2 in, 2 out]
                n257 = property on="Pre-amplification\nGain" class="Ring (strict)"("DisabledEnum"=w481) -> ()  [unwired: 2 in, 2 out]
                n258 = property on="Shutter\nClosing Time" class="DigNum (strict)"("DisabledEnum"=w481) -> ()  [unwired: 2 in, 2 out]
                n259 = property on="Horizontal\nBinning" class="DigNum (strict)"("DisabledEnum"=w481) -> ()  [unwired: 2 in, 2 out]
                n260 = property on="Vertical\nBinning" class="DigNum (strict)"("DisabledEnum"=w481) -> ()  [unwired: 2 in, 2 out]
                n261 = property on="Image\nFInal Column" class="DigNum (strict)"("DisabledEnum"=w481) -> ()  [unwired: 2 in, 2 out]
                n262 = property on="CH1on" class="Bool (strict)"("DisabledEnum"=w481) -> ()  [unwired: 2 in, 2 out]
                n263 = property on="CH2on" class="Bool (strict)"("DisabledEnum"=w481) -> ()  [unwired: 2 in, 2 out]
                n264 = property on="CH3 on" class="Bool (strict)"("DisabledEnum"=w481) -> ()  [unwired: 2 in, 2 out]
                n265 = property on="CH4 on" class="Bool (strict)"("DisabledEnum"=w481) -> ()  [unwired: 2 in, 2 out]
                n266 = property on="Image\nFinal Line" class="DigNum (strict)"("DisabledEnum"=w481) -> ()  [unwired: 2 in, 2 out]
                n267 = property on="Image\nInitial Column" class="DigNum (strict)"("DisabledEnum"=w481) -> ()  [unwired: 2 in, 2 out]
                n268 = property on="Image \nInitial Line" class="DigNum (strict)"("DisabledEnum"=w481) -> ()  [unwired: 2 in, 2 out]
              }
              frame #2 {
                n269 = Unbundle By Name(w500) -> ("Trigger Mode Status"=→"String":string, "Focus_connection"=→"Focus 160":bool, "WS_connection"=→"Weather":bool)
              }
              frame #3 {
                n270 = Unbundle By Name(w502) -> ("Trigger General Status"=→"String 2":string)
              }
              frame #4 {
                n271 = Unbundle By Name(w510) -> ("Instrument Motor error"=w503:T18, "Instrument Status"=w504:T19, "Instrument States.WPROT State"=w509:i32, "Instrument Pos Names.WPROT posname"=w508:string, "Instrument Pos Names.WPSEL posname"=w507:string, "Instrument Pos Names.CALW posname"=w506:string, "Instrument Pos Names.ASEL posname"=w505:string)
                n272 = stacked-sequence {
                  tunnel: w504 -> [w517 w522 w527 w531 w535 w540 w545 w551 w553]
                  tunnel: w509 -> [w513 _ _ _ _ _ _ _ _]
                  tunnel: w508 -> [_ w520 _ _ _ _ _ _ _]
                  tunnel: w507 -> [_ _ w525 _ _ _ _ _ _]
                  tunnel: w506 -> [_ _ _ _ _ w538 _ _ _]
                  tunnel: w505 -> [_ _ _ _ _ _ w543 _ _]
                  tunnel: w503 -> [_ w519 w524 w530 w534 w537 w542 _ _]
                  frame #0 {
                    # "Pisca quando BUSY"
                    n273 = Unbundle By Name(w517) -> ("WPROT pos"=w514:dbl)
                    "WaveplatePos 2" <- w514
                    n274 = Equal?(x=w513, y=3) -> (x = y?=w511:bool)
                    n275 = property on="WaveplatePos 2" class="DigNum (strict)"("Blinking"=w511) -> ()  [unwired: 2 in, 2 out]
                    n276 = Number To Fractional String(number=w514, precision (6)=i16 1) -> (F-format string=→"Angle":string)  [unwired: 2 in]
                  }
                  frame #1 {
                    n277 = Unbundle By Name(w519) -> ("WPROT error"=→"WPROT motor error":bool)
                    n278 = Unbundle By Name(w522) -> ("WPROT pos"=→"Position WPROT":dbl)
                    "PosName WPROT" <- w520
                  }
                  frame #2 {
                    n279 = Unbundle By Name(w527) -> ("WPSEL pos"=→"Position WPSEL":dbl)
                    n280 = Unbundle By Name(w524) -> ("WPSEL error"=→"WPSEL motor error":bool)
                    "PosName WPSEL" <- w525
                  }
                  frame #3 {
                    n281 = Unbundle By Name(w531) -> ("GMIR pos"=→"Position GMIR" →"Position GMIR 2":dbl)
                    n282 = Unbundle By Name(w530) -> ("GMIR error"=→"GMIR motor error" →"GMIR motor error 2":bool)
                  }
                  frame #4 {
                    n283 = Unbundle By Name(w535) -> ("GFOC pos"=→"Position GFOC" →"Position GFOC 2":dbl)
                    n284 = Unbundle By Name(w534) -> ("GFOC error"=→"GFOC motor error" →"GFOC motor error 2":bool)
                  }
                  frame #5 {
                    n285 = Unbundle By Name(w540) -> ("CALW pos"=→"Position CALW":dbl)
                    n286 = Unbundle By Name(w537) -> ("CALW error"=→"CALW motor error":bool)
                    "PosName CALW" <- w538
                  }
                  frame #6 {
                    n287 = Unbundle By Name(w545) -> ("ASEL pos"=→"PosName ASEL":dbl)
                    n288 = Unbundle By Name(w542) -> ("ASEL error"=→"ASEL motor error":bool)
                    "PosName ASEL" <- w543
                  }
                  frame #7 {
                    w547 = cluster{u32, u32}[] [{16711680, 16711680}, {15400704, 15400704}, {16776722, 0}, {16776722, 0}]  # amarelo
                    w546 = cluster{u32, u32}[] [{16711680, 16711680}, {6618880, 6618880}, {16776722, 0}, {16776722, 0}]  # verde
                    n289 = Unbundle By Name(w551) -> ("connection"=→"S4ICSoft":bool, "operational"=w549:bool)
                    n290 = Select(t=w546, s=w549, f=w547) -> (s? t:f=w548:cluster{u32, u32}[])
                    n291 = property on="S4ICSoft" class="Bool (strict)"("Colors [4]"=w548) -> ()  [unwired: 2 in, 2 out]
                  }
                  frame #8 {
                    n292 = Unbundle By Name(w553) -> ("String Status"=→"Status":string)
                  }
                }
              }
              frame #5 {
                n293 = Unbundle By Name(w556) -> ("Sync Box State"=→"Current State":i32, "Trigger_connection"=→"Sync Box" →"LedExtSync":bool)
              }
              frame #6 {
                # "Instrument States.<device> State\n\n0: nao fez INIT e está parado (mode = IDLE ou WAITING\n                                                    contdition = default)\n1: nao fez INIT e está movendo (mode = IDLE ou WAITING\n                                                    contdition = BUSY)\n\n2: fez INIT e está parado (mode = default)\n                                            condition = READY)\n3: fez INIT e está movendo (mode = default)\n                                            condition = BUSY)"
                n294 = Unbundle By Name(w559) -> ("Instrument States"=w558:T20, "Instrument Pos Names"=w557:T21)
                n295 = stacked-sequence {
                  tunnel: w558 -> [w567 w589 w607 w641 w670]
                  tunnel: w557 -> [w563 _ w605 w637 _]
                  frame #0 {
                    # "WPSEL"
                    n296 = Unbundle By Name(w563) -> ("WPSEL posname"=w560:string)
                    n297 = Unbundle By Name(w567) -> ("WPSEL State"=w566:i32)
                    n298 = local read "WPSEL Status"() -> (w562:bool)
                    n299 = case shown="2" w566 {
                      tunnel: [cluster{u32, u32}[] [{9868950, 9868950}, {9868950, 9868950}] ("Colors [4]") cluster{u32, u32}[] [{9868950, 9868950}, {9868950, 9868950}] ("Colors [4]") cluster{u32, u32}[] [{16318208, 16318208}, {16318208, 16318208}] ("Colors [4]") cluster{u32, u32}[] [{6618880, 2424594}, {6618880, 2424594}] ("Colors [4]") w581] -> w565
                      tunnel: [FALSE ("WPROT Status") FALSE ("WPROT Status") TRUE ("WPROT Status") FALSE ("WPROT Status") w583] -> w564
                      tunnel: w562 -> [_ _ _ _ w582]
                      tunnel: ["" "" "" w577 ""] -> w561
                      tunnel: w560 -> [_ _ _ w577 _]
                      frame Default {
                      }
                      frame 0 {
                      }
                      frame 1 {
                      }
                      frame 2 {
                      }
                      frame 3 {
                        n300 = case shown="True" w582 {
                          tunnel: [cluster{u32, u32}[] [{7563008, 7563008}, {7563008, 7563008}] ("Colors [4]") cluster{u32, u32}[] [{16318208, 16318208}, {16318208, 16318208}] ("Colors [4]")] -> w581
                          frame False {
                          }
                          frame True {
                          }
                        }
                        n301 = Not(x=w582) -> (.not. x?=w583:bool)
                      }
                    }
                    "WPSEL Status" <- w564
                    "Waveplate" <- w564
                    n302 = property on="Waveplate" class="Bool (strict)"("Colors [4]"=w565, "BoolText.Text"=w561) -> ()  [unwired: 2 in, 2 out]
                    n303 = property on="WPSEL Status" class="Bool (strict)"("Colors [4]"=w565) -> ()  [unwired: 2 in, 2 out]
                  }
                  frame #1 {
                    # "WPROT"
                    n304 = Unbundle By Name(w589) -> ("WPROT State"=w588:i32)
                    n305 = case shown="2" w588 {
                      tunnel: [cluster{u32, u32}[] [{9868950, 9868950}, {9868950, 9868950}] ("Colors [4]") cluster{u32, u32}[] [{9868950, 9868950}, {9868950, 9868950}] ("Colors [4]") cluster{u32, u32}[] [{16318208, 16318208}, {16318208, 16318208}] ("Colors [4]") cluster{u32, u32}[] [{6618880, 6618880}, {6618880, 6618880}] ("Colors [4]") cluster{u32, u32}[] [{16318208, 16318208}, {16318208, 16318208}] ("Colors [4]")] -> w587
                      tunnel: [FALSE ("WPROT Status") FALSE ("WPROT Status") TRUE ("WPROT Status") FALSE ("WPROT Status") TRUE ("WPROT Status")] -> w586
                      frame Default {
                      }
                      frame 0 {
                      }
                      frame 1 {
                      }
                      frame 2 {
                      }
                      frame 3 {
                      }
                    }
                    "WPROT Status" <- w586
                    n306 = property on="WPROT Status" class="Bool (strict)"("Colors [4]"=w587) -> ()  [unwired: 2 in, 2 out]
                  }
                  frame #2 {
                    # "CALW"
                    n307 = Unbundle By Name(w607) -> ("CALW State"=w606:i32)
                    n308 = Unbundle By Name(w605) -> ("CALW posname"=w604:string)
                    n309 = local read "CALW Status"() -> (w600:bool)
                    n310 = case shown="3" w606 {
                      tunnel: [cluster{u32, u32}[] [{9868950, 9868950}, {9868950, 9868950}] ("Colors [4]") cluster{u32, u32}[] [{9868950, 9868950}, {9868950, 9868950}] ("Colors [4]") cluster{u32, u32}[] [{16318208, 16318208}, {16318208, 16318208}] ("Colors [4]") cluster{u32, u32}[] [{6618880, 6618880}, {6618880, 6618880}] ("Colors [4]") w627] -> w601
                      tunnel: [FALSE ("WPROT Status") FALSE ("WPROT Status") TRUE ("WPROT Status") FALSE ("WPROT Status") w629] -> w603
                      tunnel: w604 -> [_ _ _ w618 _]
                      tunnel: ["" "" "" w617 ""] -> w602
                      tunnel: w600 -> [_ _ _ _ w628]
                      frame Default {
                      }
                      frame 0 {
                      }
                      frame 1 {
                      }
                      frame 2 {
                        n311 = case shown="\"SHUTTER\"" w618 {
                          tunnel: ["" "DEPOL" "POL" "OFF" "PIN" "SHT"] -> w617
                          frame Default {
                          }
                          frame "DEPOLARIZER" {
                          }
                          frame "POLARIZER" {
                          }
                          frame "OFF" {
                          }
                          frame "PINHOLE" {
                          }
                          frame "SHUTTER" {
                          }
